vi "Calculate new position.vi"(8 "error in (no error)":errorcluster, 9 "Position from motor":i32, 10 "Direction":enum8{"", "CW", "CCW"}(ring), 11 "Current position in":dbl) -> (0 "error out":errorcluster, 3 "Position out":dbl)   [LabVIEW 2020]
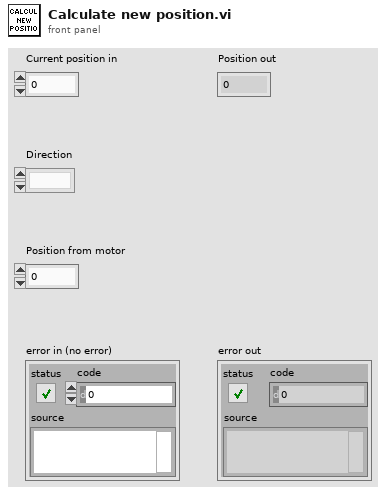
[diagram p1: front panel]
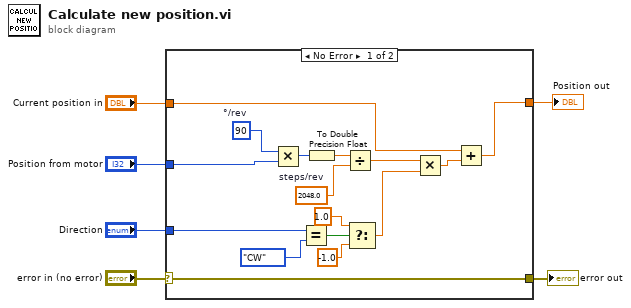
[diagram p0: block diagram]
diagram:
  n1 = case shown="No Error" "error in (no error)" {
    selector: "error in (no error)" -> [w7 w24]
    tunnel: "Direction" -> [w20 _]
    tunnel: [w19 w23] -> w5
    tunnel: "Current position in" -> [w18 w23]
    tunnel: "Position from motor" -> [w13 _]
    tunnel: [w7 w24] -> w1
    frame No Error {
      w17 = 2048.0  # steps/rev
      w14 = 90  # °/rev
      n2 = Multiply(x=w14, y=w13) -> (x*y=w15:i32)
      n3 = Equal?(x=w20, y=enum8{"", "CW", "CCW"}."CW") -> (x = y?=w22:bool)
      n4 = To Double Precision Float(number=w15) -> (double precision float=w16:dbl)
      n5 = Divide(x=w16, y=w17) -> (x/y=w9:dbl)
      n6 = Select(t=1.0, s=w22, f=-1.0) -> (s? t:f=w10:dbl)
      n7 = Multiply(x=w9, y=w10) -> (x*y=w8:dbl)
      n8 = Add(x=w18, y=w8) -> (x+y=w19:dbl)
    }
    frame Error {
    }
  }
  "Position out" <- w5
  "error out" <- w1
